vi "Error Channels Write Single.vi"(8 "error in":errorcluster, 9 "Channel Index":i32, 10 "Error Channels STS":i32, 11 "Cycler in":refnum<class "Cycler.lvclass">) -> (0 "error out":errorcluster, 3 "Cycler out":refnum<class "Cycler.lvclass">)   [LabVIEW 2023, in "Cycler.lvclass"]
uses:
  Cycler.lvclass
  Cycler.lvclass/Cycler.ctl
  Low Level Capabilities/Error Channels/Error Channels.lvclass
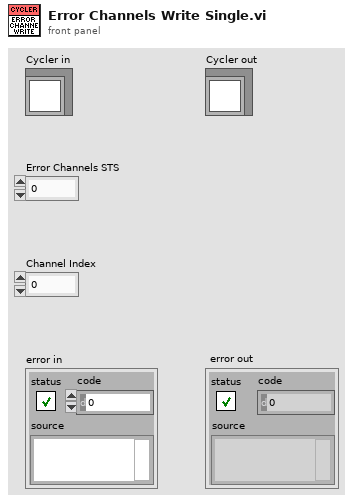
[diagram p1: front panel]
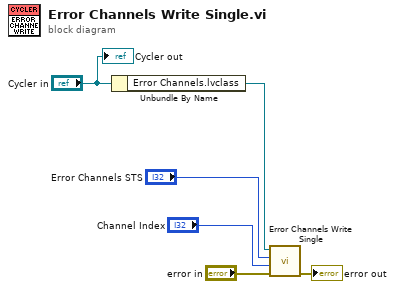
[diagram p0: block diagram]
diagram:
  n1 = Unbundle By Name("Cycler in") -> ("Error Channels.lvclass"=w5:refnum<class "Error Channels.lvclass">)
  n2 = call-dynamic "Error Channels Write Single.vi"("error in"="error in", "Channel Index"="Channel Index", "Error Channels STS"="Error Channels STS", "Error Channels in"=w5) -> ("error out"=→"error out":errorcluster)  [unwired: 6 in, 1 out]
  "Cycler out" <- "Cycler in"
